vi "25_1.vi"() -> ()   [LabVIEW 2020]
panel:
  out "x = y?":bool=TRUE
  out "Encryption Key 2":dbl=14897079.0
  out "Encryption Key 1":dbl=14897079.0
  out "Door Loop Size":i32=11
  out "Key Loop Size":i32=8
  in  "Door":dbl=7734663.0
  in  "Key":dbl=1614360.0
  in  "Door Test":dbl=17807724.0
  in  "Key Test":dbl=5764801.0
  in  "Switch":bool=TRUE
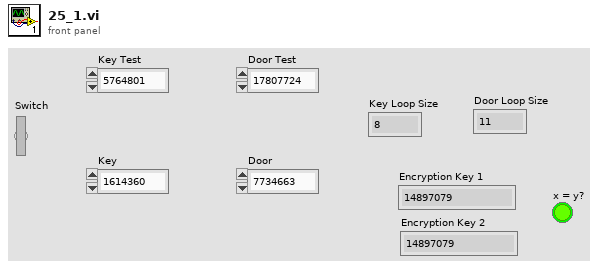
[diagram p1: front panel]
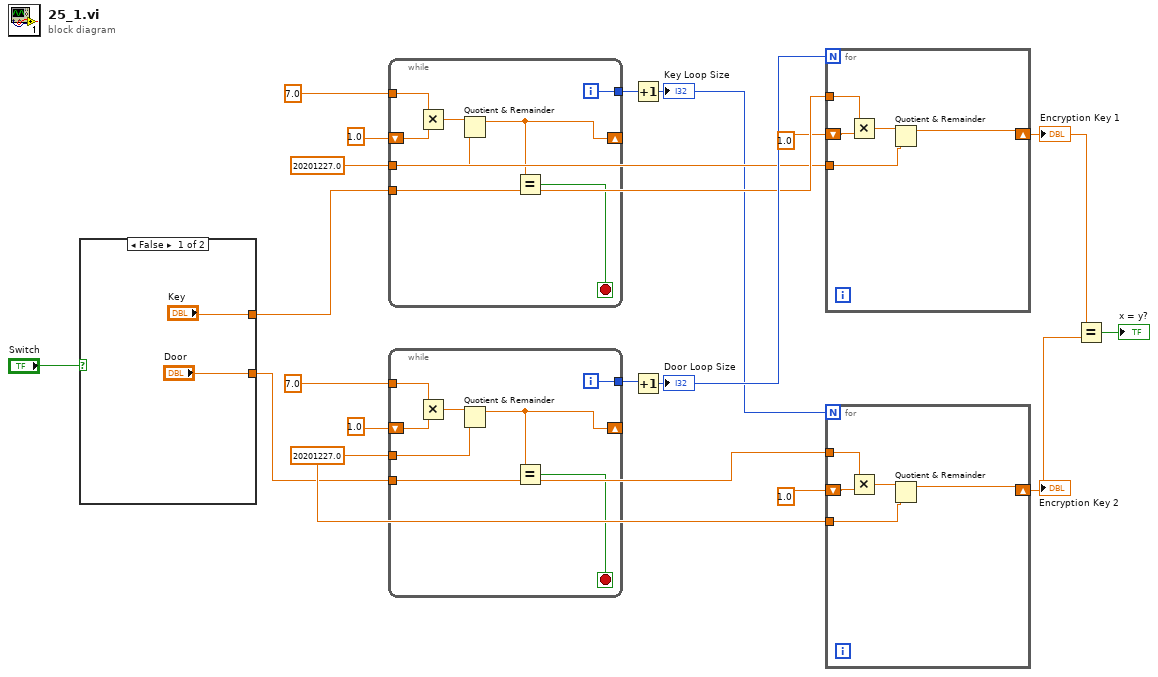
[diagram p0: block diagram]
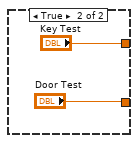
[diagram p2: hidden frame]
diagram:
  w5 = 20201227.0
  w8 = 20201227.0
  n1 = case shown="False" "Switch" {
    tunnel: ["Key" "Key Test"] -> w10
    tunnel: ["Door" "Door Test"] -> w4
    frame False {
    }
    frame True {
    }
  }
  n2 = while {
    shift-right: [w25] -> _
    shift-left: 1.0 -> [w30]
    tunnel: w10 -> [w26]
    tunnel: 7.0 -> [w29]
    tunnel: w8 -> [w27]
    tunnel: [w23] -> w15
    i -> [w23]
    stop <- w24 stop-if-true
    n3 = Multiply(x=w29, y=w30) -> (x*y=w28:dbl)
    n4 = Quotient & Remainder(x=w28, y=w27) -> (x-y*floor(x/y)=w25:dbl)  [unwired: 1 out]
    n5 = Equal?(x=w25, y=w26) -> (x = y?=w24:bool)
  }
  n6 = while {
    shift-right: [w33] -> _
    shift-left: 1.0 -> [w38]
    tunnel: w4 -> [w34]
    tunnel: 7.0 -> [w37]
    tunnel: w5 -> [w35]
    tunnel: [w31] -> w12
    i -> [w31]
    stop <- w32 stop-if-true
    n7 = Multiply(x=w37, y=w38) -> (x*y=w36:dbl)
    n8 = Quotient & Remainder(x=w36, y=w35) -> (x-y*floor(x/y)=w33:dbl)  [unwired: 1 out]
    n9 = Equal?(x=w33, y=w34) -> (x = y?=w32:bool)
  }
  n10 = Increment(x=w15) -> (x+1=w6:i32)
  "Key Loop Size" <- w6
  n11 = Increment(x=w12) -> (x+1=w11:i32)
  "Door Loop Size" <- w11
  n12 = for {
    N: w11 -> [_]
    shift-right: [w39] -> w2
    shift-left: 1.0 -> [w41]
    tunnel: w10 -> [w42]
    tunnel: w8 -> [w40]
    n13 = Multiply(x=w42, y=w41) -> (x*y=w43:dbl)
    n14 = Quotient & Remainder(x=w43, y=w40) -> (x-y*floor(x/y)=w39:dbl)  [unwired: 1 out]
  }
  "Encryption Key 1" <- w2
  n15 = for {
    N: w6 -> [_]
    shift-right: [w44] -> w3
    shift-left: 1.0 -> [w46]
    tunnel: w4 -> [w47]
    tunnel: w5 -> [w45]
    n16 = Multiply(x=w47, y=w46) -> (x*y=w48:dbl)
    n17 = Quotient & Remainder(x=w48, y=w45) -> (x-y*floor(x/y)=w44:dbl)  [unwired: 1 out]
  }
  "Encryption Key 2" <- w3
  n18 = Equal?(x=w2, y=w3) -> (x = y?=→"x = y?":bool)
